vi "Helper Action.vi"(8 "error in (no error)":errorcluster, 9 "Message Data":variant, 10 "Message":string, 11 "Thermal Chamber Controller In":refnum<class "Thermal Chamber Controller.lvclass">) -> (0 "error out":errorcluster, 1 "Exit?":bool, 2 "Loop Period [ms]":u32=1000, 3 "Thermal Chamber Controller Out":refnum<class "Thermal Chamber Controller.lvclass">)   [LabVIEW 2020, in "Thermal Chamber Controller.lvclass"]
doc: "The specific action implemented in the helper loop. Multiple different actions may be supported by using the Message and Message Data input to separate them. Any number of helper loops may run in parallell running the same or different actions. \nThe helper loop rate is controlled by the Loop Perid output of this method. \nIf this method throws an error, the helper loop will stop. The error will be sent to the error handler configured for the process. To stop it intentionally, the Stop Helper Loop.vi should be used. \nOne caveat with the helper loop is that it will have a copy of the object attributes as they were when the helper loop was started. If the attributes are updated, the helper loop will need to be restarted to refresh attributes."
uses:
  Thermal Chamber Controller.lvclass
  Thermal Chamber Controller.lvclass/Thermal Chamber Controller.ctl
  Thermal Chamber Response Simlator/Thermal Chamber Response Simlator.lvclass
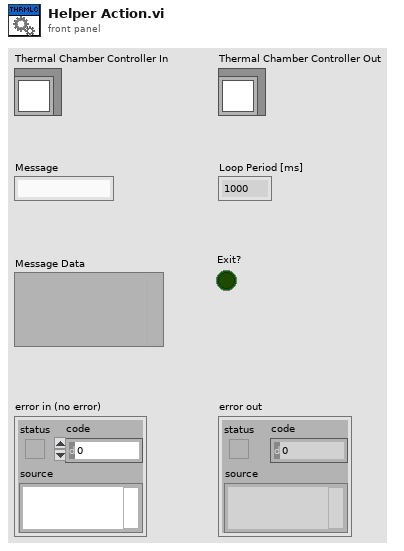
[diagram p1: front panel]
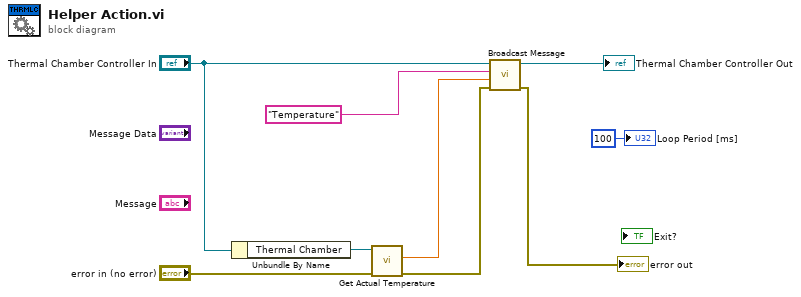
[diagram p0: block diagram]
diagram:
  n1 = Unbundle By Name("Thermal Chamber Controller In") -> ("Thermal Chamber"=w7:refnum<class "Thermal Chamber Response Simlator.lvclass">)
  n2 = call "Get Actual Temperature.vi"("error in (no error)"="error in (no error)", "Thermal Chamber Response Simlator In"=w7) -> ("error out"=w5:errorcluster, "Actual Temperature [degC]"=w4:dbl)  [unwired: 7 in, 1 out]
  n3 = call-dynamic "Broadcast Message.vi"("error in (no error)"=w5, "Message Data"=w4, "Message"="Temperature", "Process In"="Thermal Chamber Controller In") -> ("error out"=→"error out":errorcluster, "Process Out"=→"Thermal Chamber Controller Out":refnum<class "Thermal Chamber Controller.lvclass">)  [unwired: 6 in]
  "Loop Period [ms]" <- u32 100 ("Loop Period [ms]")
